vi "Open Connection.vi"(8 "Error In (no error)":errorcluster, 10 "DB Connection String/Path":string, 11 "SQLite DB Operator In":refnum<class "SQLite DB Operator.lvclass">) -> (0 "Error Out":errorcluster, 3 "SQLite DB Operator Out":refnum<class "SQLite DB Operator.lvclass">)   [LabVIEW 2023, in "SQLite DB Operator.lvclass"]
uses:
  SQLite DB Operator.lvclass
  SQLite DB Operator.lvclass/SQLite DB Operator.ctl
  <vilib>/drjdpowell/SQLite Library/SQL Connection/Open (string).vi
  <vilib>/drjdpowell/SQLite Library/SQL Connection/Connection.lvclass
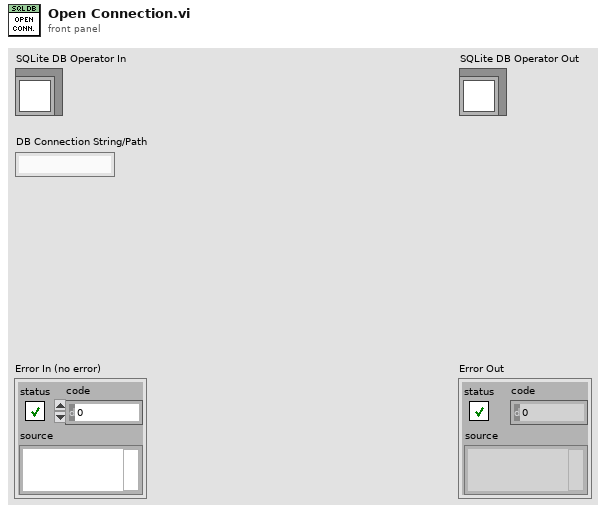
[diagram p1: front panel]
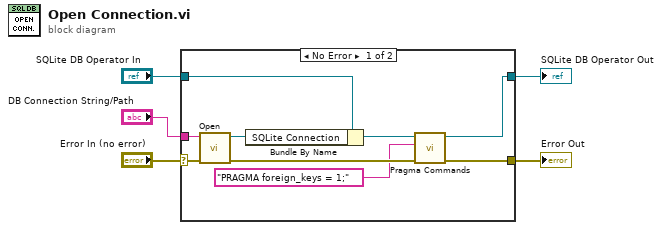
[diagram p0: block diagram]
diagram:
  n1 = case shown="No Error" "Error In (no error)" {
    selector: "Error In (no error)" -> [w13 w15]
    tunnel: [w9 w15] -> w3
    tunnel: [w8 w16] -> w4
    tunnel: "SQLite DB Operator In" -> [w14 w16]
    tunnel: "DB Connection String/Path" -> [w12 _]
    frame No Error {
      n2 = call-poly <vilib>:"Open.vi"("error in (no error)"=w13, "db file"=w12) -> ("error out"=w10:errorcluster, "SQLite Connection"=w11:refnum<class "Connection.lvclass">)  [unwired: 8 in]
      n3 = Bundle By Name(cluster=w14, "SQLite Connection"=w11) -> (w7:refnum<class "SQLite DB Operator.lvclass">)
      n4 = call "Pragma Commands.vi"("Error In (no error)"=w10, "SQL Command"="PRAGMA foreign_keys = 1;", "SQLite DB Operator In"=w7) -> ("Error Out"=w9:errorcluster, "SQLite DB Operator Out"=w8:refnum<class "SQLite DB Operator.lvclass">)  [unwired: 7 in]
    }
    frame Error {
    }
  }
  "Error Out" <- w3
  "SQLite DB Operator Out" <- w4
